vi "testItemInfoQuery.vi"(10 "testItem":string, 11 "singleItemInfo":T1[](array[typedef])) -> (2 "testResult":string, 3 "Limit":dbl[](array[numeric]))   [LabVIEW 2011]
uses:
  dataType/sSpec.ctl
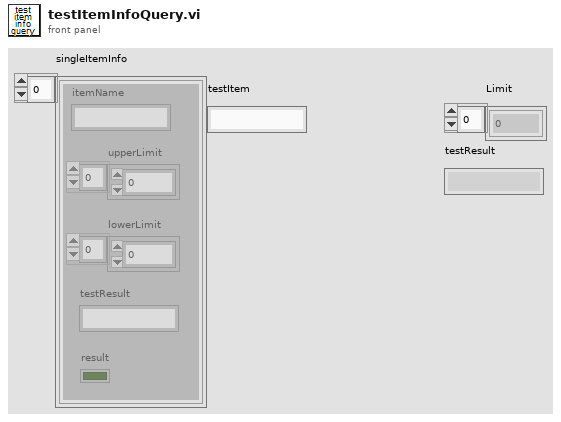
[diagram p1: front panel]
types:
  T1 = typedef "sSpec.ctl" = cluster{"itemName":string, "upperLimit":dbl[], "lowerLimit":dbl[], "testResult":string, "result":bool}
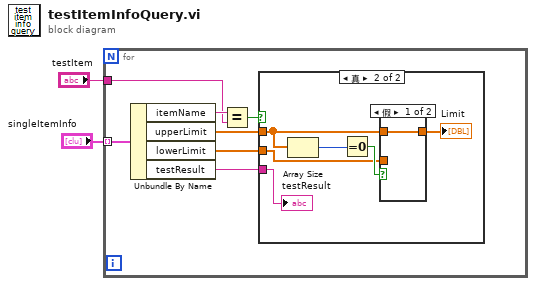
[diagram p0: block diagram]
diagram:
  n1 = for {
    tunnel: "singleItemInfo" -> [w9] mode=indexing
    tunnel: "testItem" -> [w7]
    n2 = Unbundle By Name(w9) -> ("itemName"=w8:string, "upperLimit"=w5:dbl[], "lowerLimit"=w4:dbl[], "testResult"=w3:string)
    n3 = Equal?(x=w8, y=w7) -> (x = y?=w6:bool)
    n4 = case shown="真" w6 {
      tunnel: w5 -> [_ w12]
      tunnel: w4 -> [_ w13]
      tunnel: w3 -> [_ w10]
      frame False {
      }
      frame True {
        n5 = Array Size(array=w12) -> (size(s)=w15:i32)
        n6 = Equal To 0?(x=w15) -> (x = 0?=w14:bool)
        n7 = case shown="假" w14 {
          tunnel: w13 -> [_ w17]
          tunnel: [w16 w17] -> w11
          tunnel: w12 -> [w16 _]
          frame False {
          }
          frame True {
          }
        }
        "Limit" <- w11
        "testResult" <- w10
      }
    }
  }
